vi "cameratest.vi"   [LabVIEW 2019]
uses:
  Hamamatsu_class/Hamamatsu.lvclass
types:
  T1 = typedef "IMAQ Image.ctl" = refnum<image>
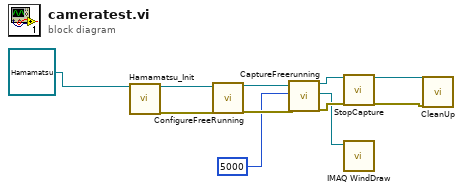
[diagram p0: block diagram]
diagram:
  n1 = call "Hamamatsu_Init.vi"("object in"=refnum<class "Hamamatsu.lvclass"> refnum ("Hamamatsu")) -> ("object out"=w10:refnum<class "Hamamatsu.lvclass">, "error out"=w6:errorcluster)  [unwired: 17 in]
  n2 = call-dynamic "ConfigureFreeRunning.vi"("object in"=w10, "error in (no error)"=w6) -> ("object out"=w9:refnum<class "Hamamatsu.lvclass">, "error out"=w5:errorcluster)  [unwired: 16 in]
  n3 = call-dynamic "CaptureFreerunning.vi"("object in"=w9, "Timeout"=5000, "error in (no error)"=w5) -> ("object out"=w8:refnum<class "Hamamatsu.lvclass">, "FreeRunningImage"=w2:T1, "error out"=w4:errorcluster)  [unwired: 13 in, 1 out]
  n4 = call-dynamic "StopCapture.vi"("object in"=w8, "error in (no error)"=w4) -> ("object out"=w7:refnum<class "Hamamatsu.lvclass">, "error out"=w3:errorcluster)  [unwired: 16 in]
  n5 = call "IMAQ WindDraw"("Image"=w2) -> ()  [unwired: 9 in, 2 out]
  n6 = call-dynamic "CleanUp.vi"("object in"=w7, "error in (no error)"=w3) -> ()  [unwired: 16 in, 2 out]
